vi "Teleop.vi"(10 "Match Info":T1={"Autonomous Elapsed Seconds"=0.0, "TeleOp Elapsed Seconds"=0.0, "Disabled Elapsed Seconds"=0.0, "Visited Autonomous"=FALSE, "Visited TeleOp"=FALSE, "Visited Disabled"=FALSE, "Autonomous Settings"={"Autonomous Style"=enum."Independent", "VI Refnum"=refnum}}, 11 "Call Context":T2) -> ()   [LabVIEW 2013]
doc: "This VI is called for each TeleOp packet received from the DS where the robot is not disabled. It is often used to read from the joysticks and update I/O or to update setpoints for timed control loops. It should complete and return within 20 milliseconds or it may miss DS packets."
uses:
  <vilib>/Rock Robotics/WPI/DriverStation/WPI_DriverStationDerivedRobotMode.ctl
  <vilib>/Rock Robotics/WPI/DriverStation/WPI_DriverStationMatch Info.ctl
  <vilib>/Rock Robotics/WPI/Joystick/WPI_JoystickRefNum Registry Get.vi
  Utilities/Invert Joystick Y Axes.vi
  Common Code/Change Detect.vi
  Common Code/Change Detect Boolean.vi
  Robot Global Data.vi
  <vilib>/Rock Robotics/WPI/Joystick/WPI_JoystickGet.vi
  <vilib>/Rock Robotics/WPI/Joystick/WPI_JoystickGetSetRefNum.vi
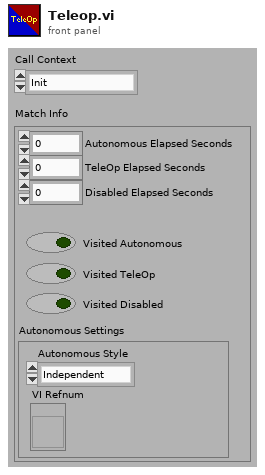
[diagram p1: front panel]
types:
  T1 = typedef "WPI_DriverStationMatch Info.ctl" = cluster{"Autonomous Elapsed Seconds":dbl, "TeleOp Elapsed Seconds":dbl, "Disabled Elapsed Seconds":dbl, "Visited Autonomous":bool, "Visited TeleOp":bool, "Visited Disabled":bool, "Autonomous Settings":cluster{"Autonomous Style":enum16{"Iterative", "Independent"}, "VI Refnum":refnum<vi>}}
  T2 = typedef "WPI_DriverStationDerivedRobotMode.ctl" = enum16{"Init", "Execute", "Stop"}
  T3 = cluster{"axis 1 (x)":dbl, "axis 2 (y)":dbl, "axis 3 (throttle)":dbl, "axis 4":dbl, "axis 5":dbl, "axis 6":dbl}
  T4 = typedef "WPI_JoystickButtonState.ctl" = cluster{"Button 1":bool, "Button 2":bool, "Button 3":bool, "Button 4":bool, "Button 5":bool, "Button 6":bool, "Button 7":bool, "Button 8":bool, "Button 9":bool, "Button 10":bool, "Button 11":bool, "Button 12":bool}
  T5 = typedef "Shooter Manual Control.ctl" = cluster{"Command":T6, "Offset":dbl, "Trigger":bool, "Add":bool, "Release":bool, "Reset":bool, "Target Pressure":dbl, "Punch":bool, "AutoPunch":bool}
  T6 = typedef "Shooter Command.ctl" = enum16{"None", "Warmup", "Shoot", "Line Shoot", "Soft Shoot", "Toss"}
  T7 = typedef "Roller Control.ctl" = cluster{"Mode":T8, "Front":enum16{"Stop", "Forward", "Reverse"}, "Back":enum16{"Stop", "Forward", "Reverse"}, "Reset":bool, "Front Piston":bool, "Halo":bool, "Net Piston":bool, "Carry Two":bool, "Hold":bool}
  T8 = typedef "Roller Mode.ctl" = enum16{"None", "Front", "Back", "Both", "Manual"}
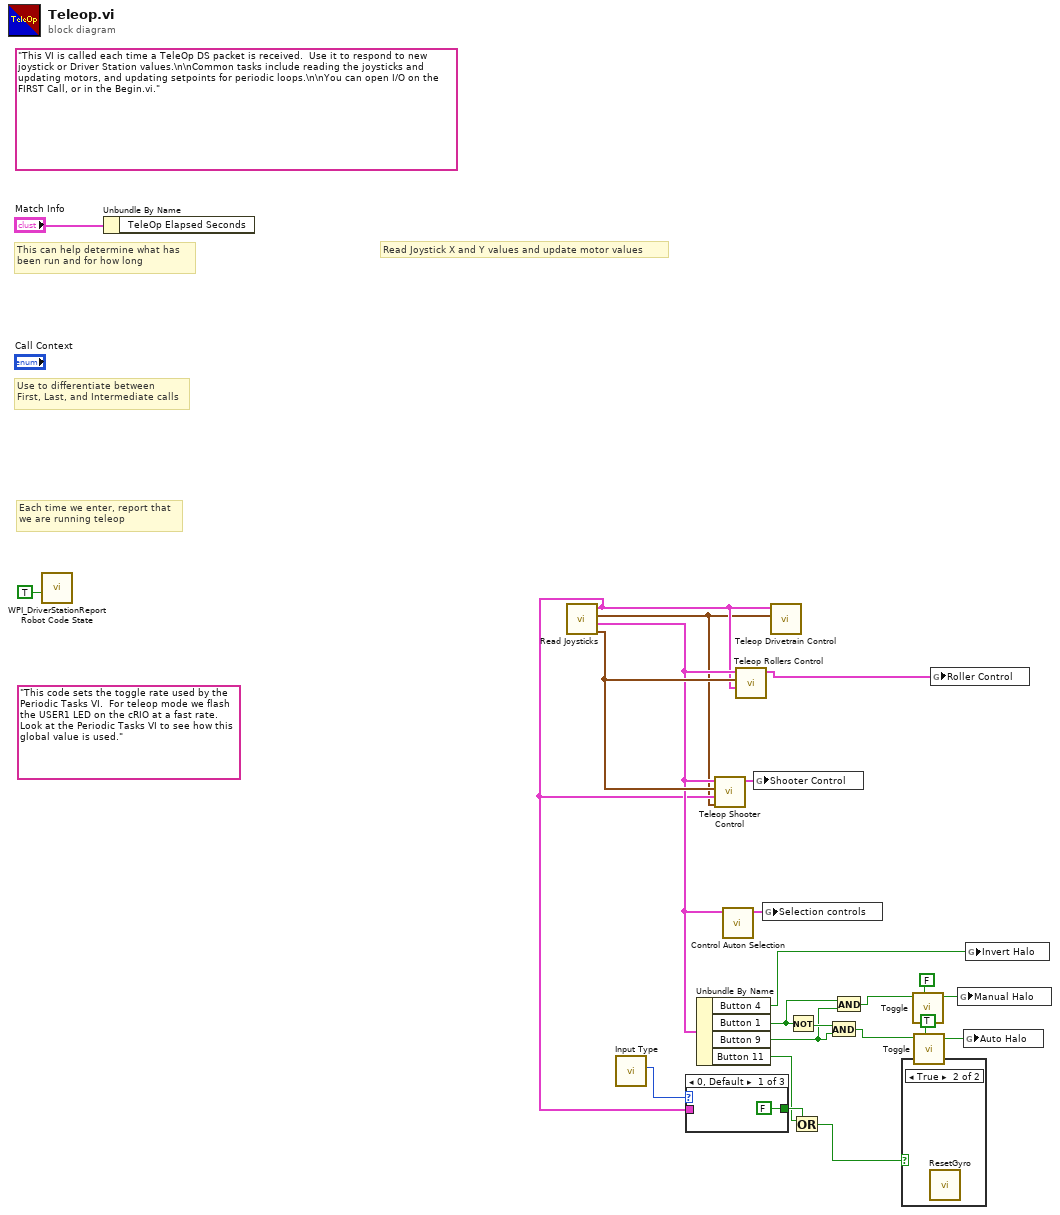
[diagram p0: block diagram]
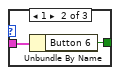
[diagram p2: hidden frame]
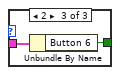
[diagram p3: hidden frame]
diagram:
  (unwired) "This code sets the toggle rate used by the Periodic Tasks VI.  For teleop mode we flash the USER1 LED on the cRIO at a fast rate.  Look at the Periodic Tasks VI to see how this global value is used."
  (unwired) "This VI is called each time a TeleOp DS packet is received.  Use it to respond to new joystick or Driver Station values.\n\nCommon tasks include reading the joysticks and updating motors, and updating setpoints for periodic loops.\n\nYou can open I/O on the FIRST Call, or in the Begin.vi."
  # "Each time we enter, report that\nwe are running teleop"
  # "Use to differentiate between\nFirst, Last, and Intermediate calls"
  # "This can help determine what has\nbeen run and for how long"
  # "Read Joystick X and Y values and update motor values"
  n1 = call <vilib>:"WPI_DriverStationReport Robot Code State.vi"("TeleOp"=TRUE ("Autonomous")) -> ()  [unwired: 10 in, 1 out]
  n2 = Unbundle By Name("Match Info") -> ()  [unwired: 1 out]
  n3 = call "Read Joysticks.vi"() -> ("Manipulator Axes"=w18:T3, "Manipulator Buttons"=w17:T4, "Driver Axes"=w1:T3, "Driver Buttons"=w16:T4)  [unwired: 8 in]
  n4 = call "Input Type.vi"() -> ("Mode"=w13:i32)  [unwired: 11 in]
  n5 = case shown="0, Default" w13 {
    tunnel: w16 -> [_ w25 w27]
    tunnel: [FALSE ("Button 6") w26 w28] -> w21
    frame 0, Default {
    }
    frame 1 {
      n6 = Unbundle By Name(w25) -> ("Button 6"=w26:bool)
    }
    frame 2 {
      n7 = Unbundle By Name(w27) -> ("Button 6"=w28:bool)
    }
  }
  n8 = Unbundle By Name(w17) -> ("Button 4"=w2:bool, "Button 1"=w3:bool, "Button 9"=w6:bool, "Button 11"=w19:bool)
  n9 = call "Teleop Shooter Control.vi"("Driver Axes"=w1, "Driver Buttons"=w16, "Manipulator Axes"=w18, "Manipulator Buttons"=w17) -> ("Shooter Control"=w14:T5)  [unwired: 7 in]
  n10 = call "Control Auton Selection.vi"("Driver Buttons"=w17) -> ("Selection controls"=w15:cluster{"Up":bool, "Down":bool})  [unwired: 10 in]
  n11 = call "Teleop Rollers Control.vi"("Driver Buttons"=w16, "Manipulator Axes"=w18, "Manipulator Buttons"=w17) -> ("Roller Command"=w11:T7)  [unwired: 8 in]
  n12 = global write "Robot Global Data.vi" "Shooter Control"(w14) -> ()
  n13 = global write "Robot Global Data.vi" "Selection controls"(w15) -> ()
  n14 = call "Teleop Drivetrain Control.vi"("Driver Axes"=w1, "Driver Buttons"=w16) -> ()  [unwired: 10 in]
  n15 = Not(x=w3) -> (.not. x?=w9:bool)
  n16 = Or(x=w19, y=w21) -> (x .or. y?=w20:bool)
  n17 = And(x=w9, y=w6) -> (x .and. y?=w8:bool)
  n18 = And(x=w3, y=w6) -> (x .and. y?=w5:bool)
  n19 = case shown="True" w20 {
    frame False {
    }
    frame True {
      n20 = call "ResetGyro.vi"() -> ()  [unwired: 12 in]
    }
  }
  n21 = call "Toggle.vi"("Initial Value"=FALSE, "In"=w5) -> ("Toggled"=w4:bool)  [unwired: 9 in]
  n22 = call "Toggle.vi"("Initial Value"=TRUE, "In"=w8) -> ("Toggled"=w10:bool)  [unwired: 9 in]
  n23 = global write "Robot Global Data.vi" "Roller Control"(w11) -> ()
  n24 = global write "Robot Global Data.vi" "Manual Halo"(w4) -> ()
  n25 = global write "Robot Global Data.vi" "Auto Halo"(w10) -> ()
  n26 = global write "Robot Global Data.vi" "Invert Halo"(w2) -> ()
